vi "Complete Service.vi"(0 "Room Service Monitor UI in":refnum<class "Room Service Monitor UI.lvclass">, 11 "error in (no error)":errorcluster) -> (4 "Room Service Monitor UI out":refnum<class "Room Service Monitor UI.lvclass">, 15 "error out":errorcluster)   [LabVIEW 2023, in "Room Service Monitor UI.lvlib" / "Room Service Monitor UI.lvclass"]
uses:
  Room Service Monitor UI.lvclass
  Room Service Monitor UI.lvclass/Room Service Monitor UI.ctl
  Room Service Monitor UI Messages/Send Complete Service Msg/Send Complete Service Msg.lvclass
  <vilib>/ActorFramework/Actor/Actor.lvclass
  C:/Users/bhaghyaraj/Trainings/NI Actor Framework/SDLC/UI Base/UI Base/UI Base.lvclass
  C:/Program Files/National Instruments/LabVIEW 2023/vi.lib/ActorFramework/Actor/Actor.lvclass
  C:/Users/bhaghyaraj/Trainings/NI Actor Framework/SDLC/Room Service Monitor UI/Room Service Monitor UI/Room Service Monitor UI.lvclass
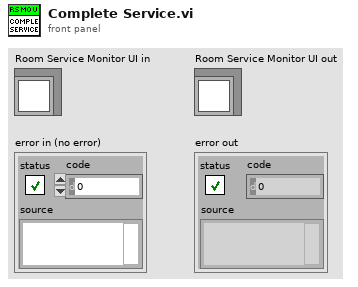
[diagram p1: front panel]
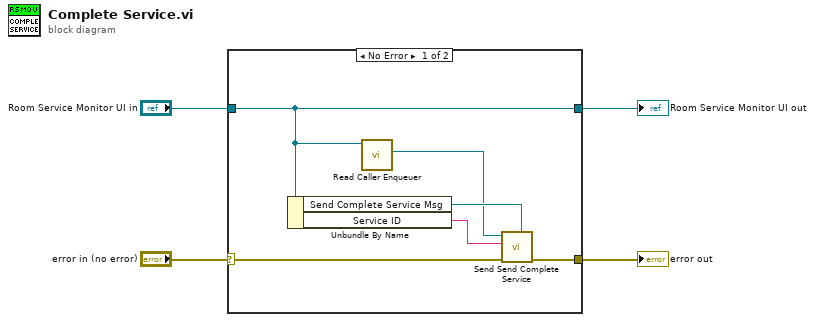
[diagram p0: block diagram]
diagram:
  n1 = case shown="No Error" "error in (no error)" {
    selector: "error in (no error)" -> [w10 w12]
    tunnel: [w9 w12] -> w3
    tunnel: [w7 w11] -> w1
    tunnel: "Room Service Monitor UI in" -> [w7 w11]
    frame No Error {
      n2 = Unbundle By Name(w7) -> ("Send Complete Service Msg"=w8:refnum<class "Send Complete Service Msg.lvclass">, "Service ID"=w5:string)
      n3 = call <vilib>:"Read Caller Enqueuer.vi"("Actor"=w7) -> ("Caller Enqueuer"=w6:refnum<class "Message Enqueuer.lvclass">)  [unwired: 10 in]
      n4 = call "Send Send Complete Service.vi"("Message Type"=w8, "error in (no error)"=w10, "Service ID"=w5, "Message Enqueuer"=w6) -> ("error out"=w9:errorcluster)  [unwired: 6 in, 1 out]
    }
    frame Error {
    }
  }
  "error out" <- w3
  "Room Service Monitor UI out" <- w1
